vi "Main.vi"(10 "Sub Panel":refnum<vi>, 11 "Module Admin":refnum<class "Delacor_lib_QMH_Module Admin.lvclass">) -> ()   [LabVIEW 2020, in "Acquisition.lvlib"]
doc: "This template is based off of the Queued Message Handler design pattern and the Queued Message Handler project template that ships with LabVIEW.\n\nThe main difference is that the queue is private to this module and communication between modules is performed via Broadcast and Request events.\n\nRequest events are wrapped in public API methods and are handled in the Event Handling Loop (EHL) of this VI. Any module can register for Broadcast events sent by this module. The EHL generates messages based on user interface actions.\n\nThe Message Handling Loop (MHL) processes messages generated by the EHL, or by other messages. The messages are string values, so new messages can be added easily to the Message Cases case structure in the MHL. Each message cluster can also provide an optional value for Message Data, which is a variant that can be converted to whatever message-specific data is required.\n_____\nBased on Delacor QMH Project Template 5.0.0.82."
uses:
  Acquisition.lvlib
  <vilib>/Delacor/Delacor QMH/Libraries/Module Admin_class/Delacor_lib_QMH_Module Admin.lvclass
  Module Data--cluster.ctl
  Start Helper Loop Argument--cluster.ctl
  Stop Helper Loop Argument--cluster.ctl
  Stop Argument--cluster.ctl
  <vilib>/Delacor/Delacor QMH/Libraries/Message Queue_class/Delacor_lib_QMH_Message Queue.lvclass/Delacor_lib_QMH_Message Queue.ctl
  <vilib>/Delacor/Delacor QMH/Libraries/Module Admin_class/Delacor_lib_QMH_Module Admin.lvclass/Delacor_lib_QMH_Module Admin.ctl
  ACQ Config Argument--cluster.ctl
  <vilib>/Utility/miscctls.llb/LVPointTypeDef.ctl
  <vilib>/Delacor/Delacor QMH/Libraries/Message Queue_class/Delacor_lib_QMH_Enqueue Message (Single).vi
  <vilib>/Delacor/Delacor QMH/Libraries/Module Admin_class/Delacor_lib_QMH_Get External Launch.vi
  <vilib>/Utility/error.llb/Error Cluster From Error Code.vi
  <vilib>/ErrorRing/Error Ring.xnode
  <vilib>/Delacor/Delacor QMH/Libraries/Message Queue_class/Delacor_lib_QMH_Message Queue.lvclass
  <vilib>/measure/NI_MABase.lvlib
panel:
  out "Waveform Graph":waveform(dbl)(graph)
  out "error out":errorcluster
  out "Status":string
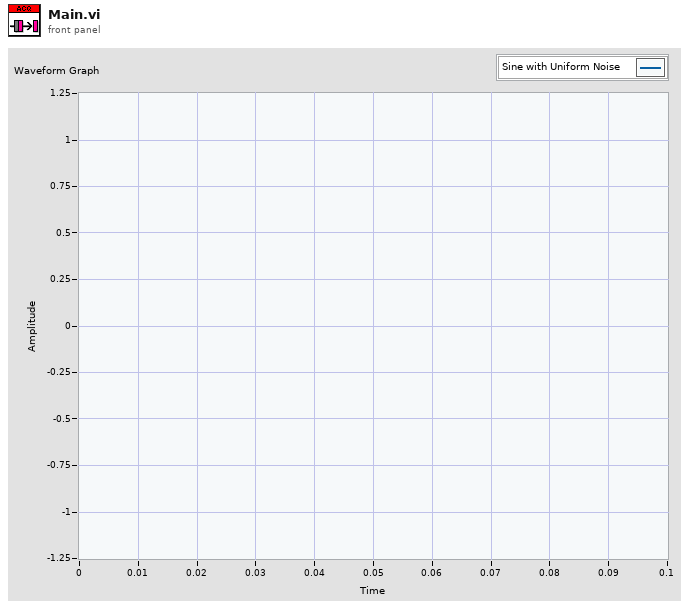
[diagram p1: front panel]
types:
  T1 = typedef "Acquisition.lvlib/Request Events--cluster.ctl" = cluster{"Stop Module":refnum<user-event>, "Show Panel":refnum<user-event>, "Hide Panel":refnum<user-event>, "Get Module Execution Status":refnum<user-event>, "Show Diagram":refnum<user-event>, "Start Helper Loop":refnum<user-event>, "Stop Helper Loop":refnum<user-event>, "ACQ Config":refnum<user-event>}
  T2 = typedef "Acquisition.lvlib/Module Data--cluster.ctl" = cluster{"Status":string}
  T3 = typedef "Acquisition.lvlib/Start Helper Loop Argument--cluster.ctl" = cluster{"DELAY Timeout":i32}
  T4 = typedef "Acquisition.lvlib/Stop Helper Loop Argument--cluster.ctl" = cluster{"Boolean":bool}
  T5 = enum32{"invalid lock state", "Not Locked", "Locked (No Password)", "Password-protected"}
  T6 = typedef "Acquisition.lvlib/Stop Argument--cluster.ctl" = cluster{"Origin":string, "Exit via Stop Module Req?":bool, "Wait for Module to stop?":bool}
  T7 = typedef "Acquisition.lvlib/ACQ Config Argument--cluster.ctl" = cluster{"Config data":cluster{"offset":dbl, "signal type":enum16{"Sine Wave", "Triangle Wave", "Square Wave", "Sawtooth Wave"}, "frequency":dbl, "amplitude":dbl, "phase":dbl, "sampling info":cluster{"Fs":dbl, "#s":dbl}, "square wave duty cycle (%)":dbl}}
  T8 = typedef "LVPointTypeDef.ctl" = cluster{"Horizontal":i16, "Vertical":i16}
  T9 = enum32{"Invalid", "Standard", "Closed", "Hidden", "Minimized", "Maximized"}
  T10 = cluster{"offset":dbl, "signal type":enum16{"Sine Wave", "Triangle Wave", "Square Wave", "Sawtooth Wave"}, "frequency":dbl, "amplitude":dbl, "phase":dbl, "sampling info":cluster{"Fs":dbl, "#s":dbl}, "square wave duty cycle (%)":dbl}
  T11 = enum16{"Sine Wave", "Triangle Wave", "Square Wave", "Sawtooth Wave"}
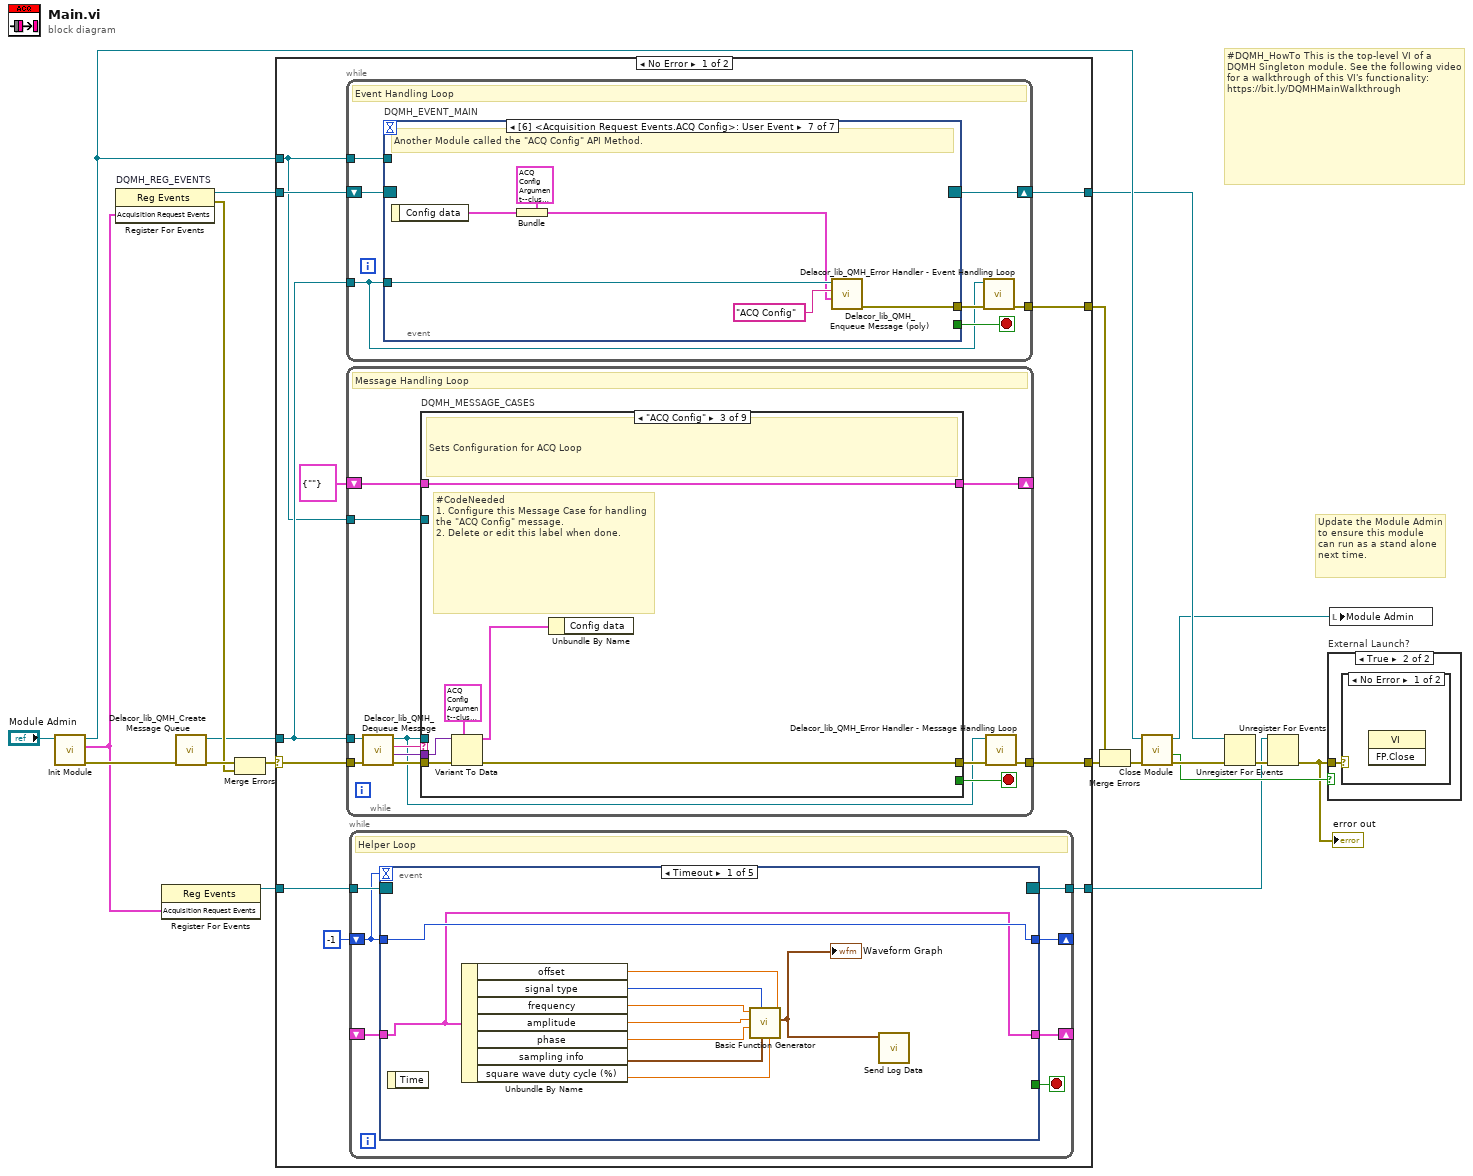
[diagram p0: block diagram]
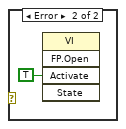
[diagram p3: hidden frame]
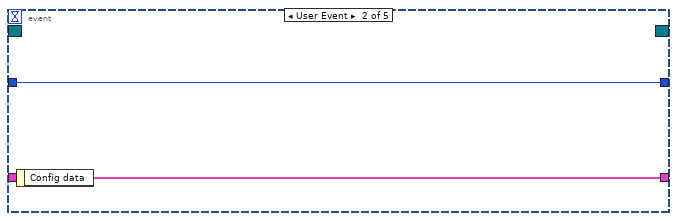
[diagram p4: hidden frame]
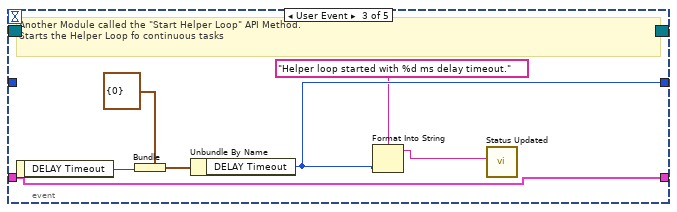
[diagram p5: hidden frame]
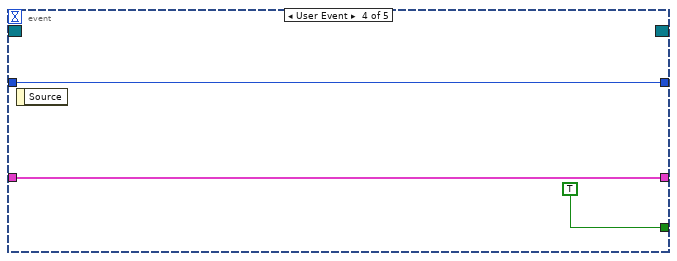
[diagram p6: hidden frame]
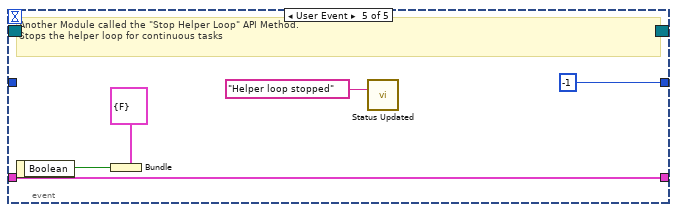
[diagram p7: hidden frame]
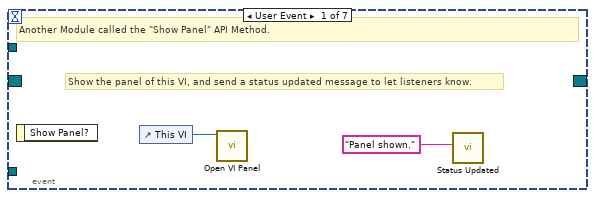
[diagram p8: hidden frame]
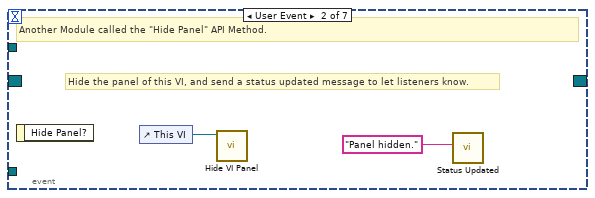
[diagram p9: hidden frame]
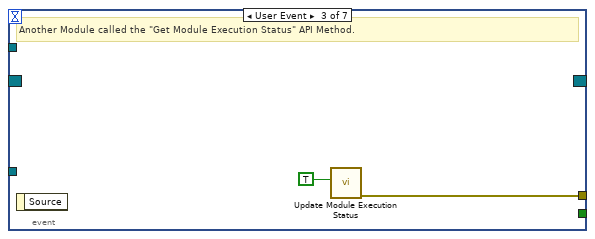
[diagram p10: hidden frame]
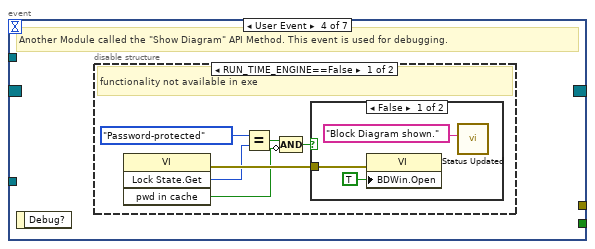
[diagram p11: hidden frame]
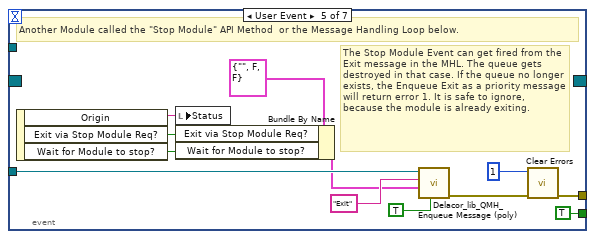
[diagram p14: hidden frame]
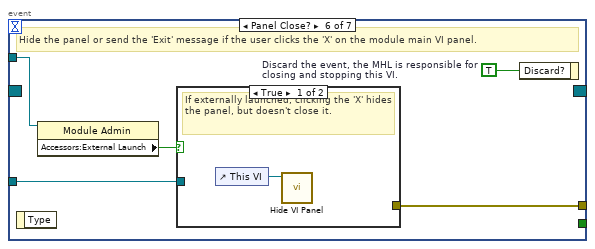
[diagram p15: hidden frame]
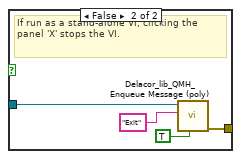
[diagram p16: hidden frame]
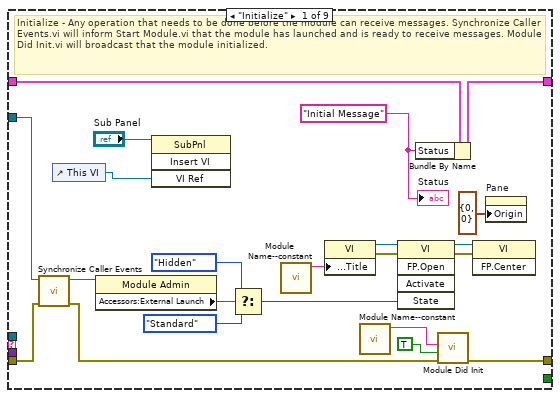
[diagram p17: hidden frame]
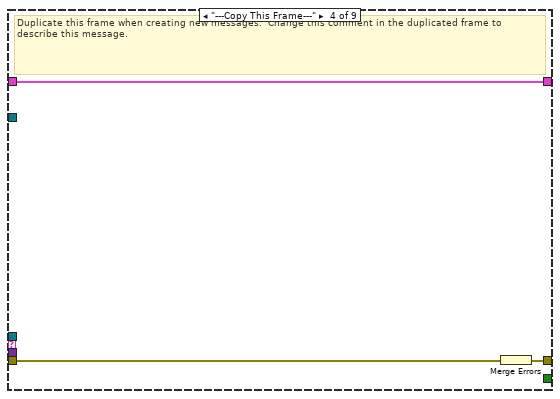
[diagram p19: hidden frame]
diagram:
  # "#DQMH_HowTo This is the top-level VI of a DQMH Singleton module. See the following video for a walkthrough of this VI's functionality: https://bit.ly/DQMHMainWalkthrough"
  # "Update the Module Admin to ensure this module can run as a stand alone next time."
  n1 = call "Init Module.vi"("Singleton Module Admin in"="Module Admin") -> ("error out"=w19:errorcluster, "Acquisition Request Events"=w3:T1, "Singleton Module Admin out"=w11:refnum<class "Delacor_lib_QMH_Module Admin.lvclass">)  [unwired: 8 in]
  n2 = register-events "DQMH_REG_EVENTS"(w3) -> (reference out=w9:refnum<event-registration>, error out=w12:errorcluster)  [unwired: 2 in]
  n3 = register-events(w3) -> (reference out=w4:refnum<event-registration>)  [unwired: 2 in, 1 out]
  n4 = call <vilib>:"Delacor_lib_QMH_Create Message Queue.vi"("error in (no error)"=w19) -> ("error out"=w14:errorcluster, "Message Queue"=w8:refnum<class "Delacor_lib_QMH_Message Queue.lvclass">)  [unwired: 9 in]
  n5 = Merge Errors(w14, w12) -> (w13:errorcluster)
  n6 = case shown="No Error" w13 {
    selector: w13 -> [w29 w224]
    tunnel: [w31 w223] -> w20
    tunnel: [w28 w229] -> w10
    tunnel: w9 -> [w26 w229]
    tunnel: w8 -> [w25 w222]
    tunnel: [w30 _] -> w17
    tunnel: w11 -> [w24 w225]
    tunnel: w4 -> [w23 w221]
    tunnel: [w22 w221] -> w1
    frame No Error {
      n7 = while {
        tunnel: w25 -> [w66]
        shift-right: [w69] -> w28
        shift-left: w26 -> [w70]
        tunnel: [w71] -> w30
        tunnel: w24 -> [w67]
        stop <- w68 stop-if-true
        # "Event Handling Loop"
        n8 = event "DQMH_EVENT_MAIN" shown="[6] <Acquisition Request Events.ACQ Config>: User Event" {
          selector: w70 -> [_ _ _ _ _ _ _]
          dyn-events: [_ _ _ _ _ _ _] -> w69
          timeout: _ -> [_ _ _ _ _ _ _]
          tunnel: [_ _ _ _ TRUE ("Discard?") _ _] -> w68
          tunnel: w66 -> [_ _ _ _ w95 w102 w115]
          tunnel: [_ _ w78 _ w98 w104 w110] -> w72
          tunnel: w67 -> [_ _ _ _ _ w101 _]
          event User Event {
            # "Show the panel of this VI, and send a status updated message to let listeners know."
            # "Another Module called the \"Show Panel\" API Method."
            n9 = event-data() -> ()  [unwired: 1 in, 1 out]
            n10 = control-ref of="This VI"() -> (w74:refnum<vi>)
            n11 = call "Open VI Panel.vi"("VI"=w74) -> ()  [unwired: 10 in, 1 out]
            n12 = call "Status Updated.vi"("Status"="Panel shown." ("format string")) -> ()  [unwired: 10 in, 1 out]
          }
          event User Event {
            # "Hide the panel of this VI, and send a status updated message to let listeners know."
            # "Another Module called the \"Hide Panel\" API Method."
            n13 = event-data() -> ()  [unwired: 1 in, 1 out]
            n14 = control-ref of="This VI"() -> (w76:refnum<vi>)
            n15 = call "Hide VI Panel.vi"("VI"=w76) -> ()  [unwired: 10 in, 1 out]
            n16 = call "Status Updated.vi"("Status"="Panel hidden." ("format string")) -> ()  [unwired: 10 in, 1 out]
          }
          event User Event {
            # "Another Module called the \"Get Module Execution Status\" API Method."
            n17 = event-data() -> ()  [unwired: 1 in, 1 out]
            n18 = call "Update Module Execution Status.vi"("Running?"=TRUE) -> ("error out"=w78:errorcluster)  [unwired: 10 in]
          }
          event User Event {
            # "Another Module called the \"Show Diagram\" API Method. This event is used for debugging."
            n19 = event-data() -> ()  [unwired: 1 in, 1 out]
            n20 = disable-structure shown="RUN_TIME_ENGINE==False" {
              frame condition #0 (active) {
                # "functionality not available in exe"
                n21 = invoke class="VI" method="Lock State.Get"() -> (error out=w84:errorcluster, "Get Lock State"=w83:T5, "pwd in cache"=w80:bool)  [unwired: 4 in, 1 out]
                n22 = Equal?(x=T5."Password-protected", y=w83) -> (x = y?=w81:bool)
                n23 = Compound Arithmetic op=AND(w81, invert w80) -> (w79:bool)
                n24 = case shown="False" w79 {
                  tunnel: w84 -> [w87 _]
                  frame False {
                    n25 = property class="VI"(error in=w87, "BDWin.Open"=TRUE ("Block Diagram Window:Open")) -> ()  [unwired: 1 in, 2 out]
                    n26 = call "Status Updated.vi"("Status"="Block Diagram shown." ("format string")) -> ()  [unwired: 10 in, 1 out]
                  }
                  frame True {
                    # "Password-protected VI, and the password is not in the cache. Do not show the diagram."
                  }
                }
              }
              frame condition #1 {
              }
            }
          }
          event User Event {
            # "The Stop Module Event can get fired from the Exit message in the MHL. The queue gets destroyed in that case. If the queue no longer exists, the Enqueue Exit as a priority message will return error 1. It is safe to ignore, because the module is already exiting."
            # "Another Module called the \"Stop Module\" API Method  or the Message Handling Loop below."
            n27 = event-data() -> ("Origin"=w94:string, "Exit via Stop Module Req?"=w90:bool, "Wait for Module to stop?"=w89:bool)  [unwired: 1 in]
            n28 = local write "Status"(w94) -> ()
            n29 = Bundle By Name(cluster=T6 {"Origin"="", "Exit via Stop Module Req?"=FALSE, "Wait for Module to stop?"=FALSE} ("Stop Argument"), "Exit via Stop Module Req?"=w90, "Wait for Module to stop?"=w89) -> (w88:T6)
            n30 = call-poly <vilib>:"Delacor_lib_QMH_Enqueue Message (poly).vi"("Priority Message? (F)"=TRUE, "Message Data"=w88, "Message"="Exit", "Message Queue in"=w95) -> ("error out"=w99:errorcluster)  [unwired: 6 in, 1 out]
            n31 = call <vilib>:"Clear Errors.vi"("error in (no error)"=w99, "specific error code to clear (0: all)"=1) -> ("error out"=w98:errorcluster)  [unwired: 4 in, 1 out]
          }
          event Panel Close? {
            w103 = TRUE  # Discard the event, the MHL is responsible for closing and stopping this VI.
            # "Hide the panel or send the 'Exit' message if the user clicks the 'X' on the module main VI panel."
            n32 = event-data() -> ()  [unwired: 1 in, 1 out]
            n33 = property class="Module Admin"(reference=w101) -> ("Accessors:External Launch"=w100:bool)  [unwired: 1 in, 2 out]
            n34 = case shown="True" w100 {
              tunnel: w102 -> [_ w108]
              tunnel: [_ w109] -> w104
              frame True {
                # "If externally launched, clicking the 'X' hides the panel, but doesn't close it."
                n35 = control-ref of="This VI"() -> (w105:refnum<vi>)
                n36 = call "Hide VI Panel.vi"("VI"=w105) -> ()  [unwired: 10 in, 1 out]
              }
              frame False {
                # "If run as a stand-alone VI, clicking the panel 'X' stops the VI."
                n37 = call-poly <vilib>:"Delacor_lib_QMH_Enqueue Message (poly).vi"("Priority Message? (F)"=TRUE, "Message"="Exit", "Message Queue in"=w108) -> ("error out"=w109:errorcluster)  [unwired: 7 in, 1 out]
              }
            }
            n38 = event-data("Discard?"=w103) -> ()  [unwired: 1 in, 1 out]
          }
          event User Event {
            # "Another Module called the \"ACQ Config\" API Method."
            n39 = event-data() -> ("Config data"=w111:T10)  [unwired: 1 in]
            n40 = Bundle(cluster=T7 {"Config data"={"offset"=0.0, "signal type"=enum."Sine Wave", "frequency"=10.0, "amplitude"=1.0, "phase"=0.0, "sampling info"={"Fs"=1000.0, "#s"=1000.0}, "square wave duty cycle (%)"=50.0}} ("ACQ Config Argument"), "Config data"=w111) -> (w112:T7)
            n41 = call-poly <vilib>:"Delacor_lib_QMH_Enqueue Message (poly).vi"("Message Data"=w112, "Message"="ACQ Config", "Message Queue in"=w115) -> ("error out"=w110:errorcluster)  [unwired: 7 in, 1 out]
          }
        }
        n42 = call-dynamic "Delacor_lib_QMH_Error Handler - Event Handling Loop.vi"("error in (no error)"=w72, "Message Queue in"=w66) -> ("dup error in"=w71:errorcluster)  [unwired: 8 in, 1 out]
      }
      n43 = while {
        tunnel: w25 -> [w118]
        shift-right: [w122] -> _
        shift-left: T2 {"Status"=""} ("Data Cluster") -> [w123]
        tunnel: w29 -> [w126]
        tunnel: [w124] -> w31
        tunnel: w24 -> [w116]
        stop <- w121 stop-if-true
        # "Message Handling Loop"
        n44 = call-dynamic "Delacor_lib_QMH_Dequeue Message.vi"("error in (no error)"=w126, "Message Queue in"=w118) -> ("error out"=w125:errorcluster, "Message Data"=w119:variant, "Message"=w120:string, "Message Queue out"=w117:refnum<class "Delacor_lib_QMH_Message Queue.lvclass">)  [unwired: 6 in]
        n45 = case "DQMH_MESSAGE_CASES" shown="\"ACQ Config\"" w120 {
          selector: w120 -> [_ _ _ _ _ _ _ _ w208]
          tunnel: w117 -> [_ _ _ _ _ _ w178 w200 _]
          tunnel: w125 -> [w147 w151 w157 w160 w162 w167 w185 w206 w210]
          tunnel: [w145 w151 w155 w159 w162 w166 w181 w203 w211] -> w127
          tunnel: w123 -> [w136 w150 w156 w158 w161 w164 w180 w199 w209]
          tunnel: [w135 w150 w156 w158 w161 w164 w180 w199 w209] -> w122
          tunnel: [_ _ _ _ _ _ _ w198 _] -> w121
          tunnel: w119 -> [_ _ w154 _ _ _ w179 w197 _]
          tunnel: w116 -> [w137 _ _ _ _ _ w177 w192 _]
          frame "Initialize" {
            w130 = "Initial Message" ("Initial Message")
            # "Initialize - Any operation that needs to be done before the module can receive messages. Synchronize Caller Events.vi will inform Start Module.vi that the module has launched and is ready to receive messages. Module Did Init.vi will broadcast that the module initialized."
            n46 = call "Synchronize Caller Events.vi"("error in (no error)"=w147, "Singleton Module Admin in"=w137) -> ("error out"=w146:errorcluster, "Singleton Module Admin out"=w132:refnum<class "Delacor_lib_QMH_Module Admin.lvclass">)  [unwired: 8 in]
            n47 = control-ref of="This VI"() -> (w128:refnum<vi>)
            n48 = property class="Module Admin"(reference=w132) -> ("Accessors:External Launch"=w141:bool)  [unwired: 1 in, 2 out]
            n49 = invoke class="SubPnl" method="Insert VI"(reference="Sub Panel", "VI Ref"=w128) -> ()  [unwired: 2 in, 4 out]
            n50 = Select(t=T9."Hidden" ("State"), s=w141, f=T9."Standard" ("State")) -> (s? t:f=w138:T9)
            n51 = call "Module Name--constant.vi"() -> ("Module Name"=w144:string)  [unwired: 11 in]
            n52 = property class="VI"("Front Panel.Title"=w144) -> (reference out=w143:refnum<vi>, error out=w149:errorcluster)  [unwired: 2 in]
            n53 = call "Module Name--constant.vi"() -> ("Module Name"=w133:string)  [unwired: 11 in]
            n54 = invoke class="VI" method="FP.Open"(reference=w143, error in=w149, "State"=w138) -> (reference out=w142:refnum<vi>, error out=w148:errorcluster)  [unwired: 2 in, 3 out]
            n55 = Bundle By Name(cluster=w136, "Status"=w130) -> (w135:T2)
            n56 = call "Module Did Init.vi"("error in (no error)"=w146, "Initialized?"=TRUE, "Origin"=w133) -> ("error out"=w145:errorcluster)  [unwired: 8 in]
            n57 = invoke class="VI" method="FP.Center"(reference=w142, error in=w148) -> ()  [unwired: 1 in, 3 out]
            n58 = property on="Pane" class="Pane"("Origin"=T8 {"Horizontal"=0, "Vertical"=0}) -> ()  [unwired: 2 in, 2 out]
            "Status" <- w130
          }
          frame "--- Module Specific ---" {
            # "Separator -- The following cases handle messages specific to this Module."
          }
          frame "ACQ Config" {
            # "#CodeNeeded\n1. Configure this Message Case for handling the \"ACQ Config\" message.\n2. Delete or edit this label when done."
            # "Sets Configuration for ACQ Loop"
            n59 = Variant To Data(error in=w157, type=T7 {"Config data"={"offset"=0.0, "signal type"=enum."Sine Wave", "frequency"=10.0, "amplitude"=1.0, "phase"=0.0, "sampling info"={"Fs"=1000.0, "#s"=1000.0}, "square wave duty cycle (%)"=50.0}} ("ACQ Config Argument"), Variant=w154) -> (data=w152:T7, error out=w155:errorcluster)
            n60 = Unbundle By Name(w152) -> ()  [unwired: 1 out]
          }
          frame "---Copy This Frame---" {
            # "Duplicate this frame when creating new messages.  Change this comment in the duplicated frame to describe this message."
            n61 = Merge Errors(w160) -> (w159:errorcluster)
          }
          frame "--- Exit and Error Handling---" {
            # "Separator - The following cases handle errors and exit messages."
          }
          frame "Simulate MHL Error" {
            # "#DQMH_HowTo The 'Simulate MHL Error' button  illustrates how the MHL handles errors. This event is instructional in nature and can be removed."
            # "Simulate an error occurring at the MHL"
            n62 = call "Module Name--constant.vi"() -> ("Module Name"=w163:string)  [unwired: 11 in]
            n63 = xnode "Error Ring"("parameter 0"=w163) -> ("error out"=w165:errorcluster)
            n64 = Merge Errors(w167, w165) -> (w166:errorcluster)
          }
          frame "Error" {
            # "#CodeRecommended - If you ever change the name of this \"Error\" message, you'll need to update the name in the Check Loop Error.vi as well."
            # "#CodeRecommended - If the module is running in standalone mode (External Launch = FALSE), this code will pop up an error dialog and call the 'Exit' message if an error occurs. Add more fine-grained error handling here."
            # "Error - Check the error message data and respond accordingly. This message is sent by the \"Error Handler\" VIs at the end of each loop in this application."
            n65 = property class="Module Admin"(reference=w177) -> ("Accessors:External Launch"=w176:bool)  [unwired: 1 in, 2 out]
            n66 = Variant To Data(error in=w185, type=errorcluster {"status"=FALSE, "code"=0, "source"=""} ("error constant"), Variant=w179) -> (data=w186:errorcluster, error out=w183:errorcluster)
            n67 = call "Module Name--constant.vi"() -> ("Module Name"=w175:string)  [unwired: 11 in]
            n68 = call "Error Reported.vi"("Additional Information"=w175, "Error"=w186) -> ()  [unwired: 9 in, 1 out]
            n69 = case shown="False" w176 {
              tunnel: [w191 _] -> w182
              tunnel: w178 -> [w189 _]
              tunnel: w186 -> [w190 _]
              frame False {
                # "If the module is running standalone, then pop up an error dialog and call the \"Exit\" message."
                n70 = call <vilib>:"Simple Error Handler.vi"("error in (no error)"=w190) -> ()  [unwired: 4 in, 5 out]
                n71 = call-poly <vilib>:"Delacor_lib_QMH_Enqueue Message (poly).vi"("Priority Message? (F)"=TRUE, "Message"="Exit", "Message Queue in"=w189) -> ("error out"=w191:errorcluster)  [unwired: 7 in, 1 out]
              }
              frame True {
                # "If the module was launched externally, calling the Error Reported broadcast VI is the only action performed by the \"Error\" message. The module's caller can then process the error appropriately."
              }
            }
            n72 = Merge Errors(w183, w182) -> (w181:errorcluster)
            n73 = local write "error out"(w181) -> ()
          }
          frame "Exit" {
            w196 = 91  # 91: not all Exit messages will have an argument
            w198 = TRUE  # Stop the VI
            # "Release the message queue reference"
            # "#CodeNeeded - Add any required cleanup code here"
            # "Exit - Exit the application."
            n74 = Variant To Data(error in=w206, type=T6 {"Origin"="", "Exit via Stop Module Req?"=FALSE, "Wait for Module to stop?"=FALSE} ("Stop Argument"), Variant=w197) -> (data=w194:T6, error out=w202:errorcluster)
            n75 = call <vilib>:"Clear Errors.vi"("error in (no error)"=w202, "specific error code to clear (0: all)"=w196) -> ("error out"=w205:errorcluster)  [unwired: 4 in, 1 out]
            n76 = control-ref of="This VI"() -> (w193:refnum<vi>)
            n77 = call-dynamic "Delacor_lib_QMH_Release Message Queue.vi"("error in (no error)"=w205, "Message Queue"=w200) -> ("error out"=w204:errorcluster)  [unwired: 9 in]
            n78 = call "Handle Exit.vi"("Stop Argument"=w194, "Admin in"=w192, "VI reference"=w193) -> ("error out"=w201:errorcluster)  [unwired: 7 in, 1 out]
            n79 = Merge Errors(w204, w201) -> (w203:errorcluster)
          }
          frame Default {
            # "'Default' case only runs if there is a message that isn't defined in any of the other cases.  Output a programming error."
            n80 = call "Module Name--constant.vi"() -> ("Module Name"=w207:string)  [unwired: 11 in]
            n81 = xnode "Error Ring"("parameter 0"=w208, "parameter 1"=w207) -> ("error out"=w212:errorcluster)
            n82 = Merge Errors(w210, w212) -> (w211:errorcluster)
          }
        }
        n83 = call-dynamic "Delacor_lib_QMH_Error Handler - Message Handling Loop.vi"("error in (no error)"=w127, "Message Queue in"=w117) -> ("dup error in"=w124:errorcluster)  [unwired: 8 in, 1 out]
      }
      n84 = while {
        tunnel: w23 -> [w38]
        tunnel: [w37] -> w22
        shift-right: [w36] -> _
        shift-left: -1 -> [w35]
        shift-right: [w33] -> _
        shift-left: _ -> [w32]
        stop <- w34 stop-if-true
        # "Helper Loop"
        n85 = event shown="[0] Timeout" {
          selector: w38 -> [_ _ _ _ _]
          dyn-events: [_ _ _ _ _] -> w37
          timeout: w35 -> [_ _ _ _ _]
          tunnel: [w48 w49 w53 w60 -1] -> w36
          tunnel: w35 -> [w48 w49 _ w60 _]
          tunnel: [_ _ _ TRUE _] -> w34
          tunnel: [w40 w50 w51 w58 w61] -> w33
          tunnel: w32 -> [w40 _ w51 w58 w61]
          event Timeout {
            n86 = event-data() -> ()  [unwired: 1 in, 1 out]
            n87 = Unbundle By Name(w40) -> ("offset"=w47:dbl, "signal type"=w46:T11, "frequency"=w45:dbl, "amplitude"=w44:dbl, "phase"=w43:dbl, "sampling info"=w42:cluster{"Fs":dbl, "#s":dbl}, "square wave duty cycle (%)"=w41:dbl)
            n88 = call <vilib>:"Basic Function Generator.vi"("offset"=w47, "square wave duty cycle (%)"=w41, "sampling info"=w42, "signal type"=w46, "phase"=w43, "amplitude"=w44, "frequency"=w45) -> ("signal out"=w39:waveform(dbl))  [unwired: 2 in, 2 out]
            "Waveform Graph" <- w39
            n89 = call "Send Log Data.vi"("signal in"=w39) -> ()  [unwired: 10 in, 1 out]
          }
          event User Event {
            n90 = event-data() -> ("Config data"=w50:T10)  [unwired: 1 in]
          }
          event User Event {
            # "Another Module called the \"Start Helper Loop\" API Method.\nStarts the Helper Loop fo continuous tasks"
            n91 = event-data() -> ("DELAY Timeout"=w56:i32)  [unwired: 1 in]
            n92 = Bundle(cluster=T3 {"DELAY Timeout"=0} ("Start Helper Loop Argument"), "DELAY Timeout"=w56) -> (w55:T3)
            n93 = Unbundle By Name(w55) -> ("DELAY Timeout"=w53:i32)
            n94 = Format Into String(format string="Helper loop started with %d ms delay timeout.", w53) -> (resulting string=w54:string)  [unwired: 2 in, 1 out]
            n95 = call "Status Updated.vi"("Status"=w54) -> ()  [unwired: 10 in, 1 out]
          }
          event User Event {
            n96 = event-data() -> ()  [unwired: 1 in, 1 out]
          }
          event User Event {
            # "Another Module called the \"Stop Helper Loop\" API Method.\nStops the helper loop for continuous tasks"
            n97 = event-data() -> ("Boolean"=w64:bool)  [unwired: 1 in]
            n98 = Bundle(cluster=T4 {"Boolean"=FALSE} ("Stop Helper Loop Argument"), "Boolean"=w64) -> ()  [unwired: 1 out]
            n99 = call "Status Updated.vi"("Status"="Helper loop stopped") -> ()  [unwired: 10 in, 1 out]
          }
        }
      }
    }
    frame Error {
      # "Synchronize Caller Events.vi will inform Start Module.vi that the module has launched and will let the code calling Start Module.vi register for broadcasts and would permit the caller receive the broadcast that an error occurred at launch time."
      n100 = call-dynamic "Delacor_lib_QMH_Release Message Queue.vi"("error in (no error)"=w224, "Message Queue"=w222) -> ("error out"=w223:errorcluster)  [unwired: 9 in]
      n101 = call "Synchronize Caller Events.vi"("Singleton Module Admin in"=w225) -> ("error out"=w230:errorcluster)  [unwired: 9 in, 1 out]
      n102 = call "Module Name--constant.vi"() -> ("Module Name"=w228:string)  [unwired: 11 in]
      n103 = Format Into String(format string="An error occurred during initialization. %s is no longer running.", w228) -> (resulting string=w226:string)  [unwired: 2 in, 1 out]
      n104 = Merge Errors(w223, w230) -> (w231:errorcluster)
      n105 = call "Error Reported.vi"("Additional Information"=w226, "Error"=w231) -> ()  [unwired: 9 in, 1 out]
    }
  }
  n106 = Merge Errors(w17, w20) -> (w16:errorcluster)
  n107 = call "Close Module.vi"("error in (no error)"=w16, "Module Admin in"=w11) -> ("error out"=w18:errorcluster, "External Launch"=w5:bool, "Module Admin out"=w6:refnum<class "Delacor_lib_QMH_Module Admin.lvclass">)  [unwired: 7 in]
  n108 = Unregister For Events(event registration refnum=w10, error in=w18) -> (error out=w15:errorcluster)
  n109 = Unregister For Events(event registration refnum=w1, error in=w15) -> (error out=w2:errorcluster)
  "error out" <- w2
  n110 = case "External Launch?" shown="True" w5 {
    tunnel: w2 -> [_ w232]
    frame False {
    }
    frame True {
      n111 = case shown="No Error" w232 {
        frame No Error {
          n112 = invoke class="VI" method="FP.Close"() -> ()  [unwired: 3 in, 3 out]
        }
        frame Error {
          n113 = invoke class="VI" method="FP.Open"("Activate"=TRUE ("Activate?")) -> ()  [unwired: 4 in, 5 out]
        }
      }
    }
  }
  n114 = local write "Module Admin"(w6) -> ()
